vi "Build path.vi"(1 "Relative path":string, 2 "Base path":string) -> (0 "Resulting path":string)   [LabVIEW 2015, in "RT Management.lvlib" / "File Transfer Behavior.lvclass"]
doc: "Builds a path up from base and relative path. This VI handles the formatting of the paths, so that they are always returned as valid paths.\n\nFor example, if the base path is \"C:\\directory\\folder\\\" and the relative path is \"/path/file/\", the resulting path would be \"/directory/folder/path/file\"."
uses:
  File Transfer Behavior.lvclass
  <vilib>/Utility/error.llb/Trim Whitespace.vi
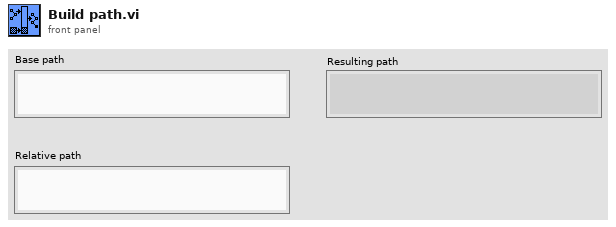
[diagram p1: front panel]
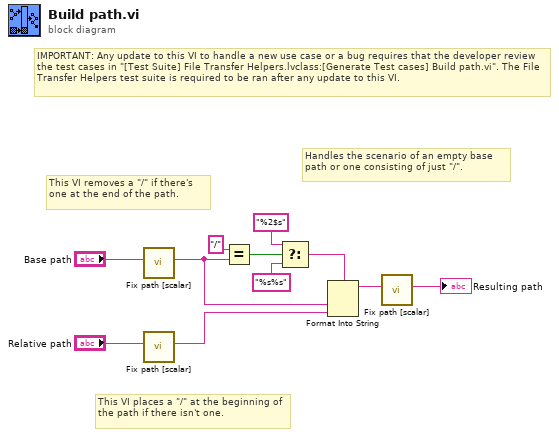
[diagram p0: block diagram]
diagram:
  # "Handles the scenario of an empty base path or one consisting of just \"/\"."
  # "IMPORTANT: Any update to this VI to handle a new use case or a bug requires that the developer review the test cases in \"[Test Suite] File Transfer Helpers.lvclass:[Generate Test cases] Build path.vi\". The File Transfer Helpers test suite is required to be ran after any update to this VI."
  # "This VI places a \"/\" at the beginning of the path if there isn't one."
  # "This VI removes a \"/\" if there's one at the end of the path."
  n1 = call "Fix path [scalar].vi"("Path in"="Base path") -> ("Path out"=w5:string)  [unwired: 8 in, 2 out]
  n2 = call "Fix path [scalar].vi"("Path in"="Relative path") -> ("Path out"=w4:string)  [unwired: 8 in, 2 out]
  n3 = Equal?(x="/", y=w5) -> (x = y?=w8:bool)
  n4 = Select(t="%2$s" ("format string"), s=w8, f="%s%s" ("format string")) -> (s? t:f=w1:string)
  n5 = Format Into String(format string=w1, w5, w4) -> (resulting string=w3:string)  [unwired: 2 in, 1 out]
  n6 = call "Fix path [scalar].vi"("Path in"=w3) -> ("Path out"=→"Resulting path":string)  [unwired: 8 in, 2 out]
